vi "GetTrigger.vi"(7 "ModuleID":i32, 8 "error in (no error)":errorcluster, 11 "ScopePluginsBase in":refnum<class "ScopePluginsBase.lvclass">) -> (0 "error out":errorcluster, 3 "ScopePluginsBase out":refnum<class "ScopePluginsBase.lvclass">)   [LabVIEW 2018, in "ScopePlugins.lvlib" / "ScopePluginsBase.lvclass"]
uses:
  ScopePluginsBase.lvclass
  ScopePlugins.lvlib
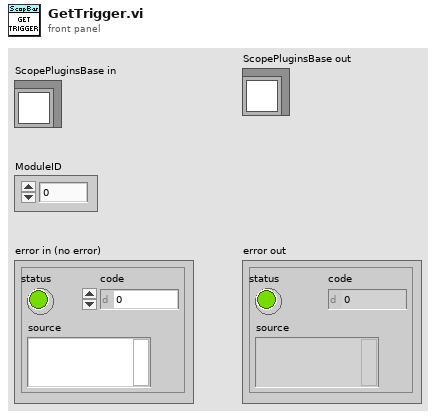
[diagram p1: front panel]
types:
  T1 = typedef "ScopePlugins.lvlib/ScopePluginsBase.lvclass/TriggerSettings.ctl" = cluster{"Common Trigger Settings":cluster{"Trigger Delay":dbl, "Reference Position":dbl, "Trigger Modifier":i32, "Auto Triggered":bool}, "Specific Trigger Settings":cluster{"Source":string, "Holdoff":dbl, "Level":dbl, "Trigger Slope":enum16{"Negative", "Positive"}, "Type":enum16{"Immediate", "Edge", "Digitial", "Window", "Hysteresis", "Width", "Runt", "Glitch", "TV", "AC Line"}, "Window Mode":i32, "Low Level":dbl, "High Level":dbl, "Coupling":u16, "Hysteresis":dbl}}
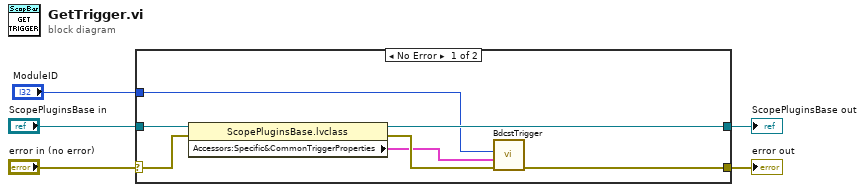
[diagram p0: block diagram]
diagram:
  n1 = case shown="No Error" "error in (no error)" {
    selector: "error in (no error)" -> [w9 w14]
    tunnel: [w7 w14] -> w4
    tunnel: [w11 w13] -> w2
    tunnel: "ScopePluginsBase in" -> [w12 w13]
    tunnel: "ModuleID" -> [w10 _]
    frame No Error {
      n2 = property class="ScopePluginsBase.lvclass"(reference=w12, error in=w9) -> (reference out=w11:refnum<class "ScopePluginsBase.lvclass">, error out=w8:errorcluster, "Accessors:Specific&CommonTriggerProperties"=w6:T1)
      n3 = call "BdcstTrigger.vi"("error in (no error)"=w8, "Specific&CommonTriggerProperties"=w6, "ModuleID"=w10) -> ("error out"=w7:errorcluster)  [unwired: 8 in]
    }
    frame Error {
    }
  }
  "error out" <- w4
  "ScopePluginsBase out" <- w2
